vi "SP Handle Data Memory Enabling.vi"(7 "Memory Exists?":bool[](array[boolean]), 9 "CH Controls":T1[](array[typedef]) {"Reference" format="%#.2g"; "Display Data" items=["Data", "Memory", "Data/Memory"]; "Format" items=["Log Mag", "Phase", "Expanded Phase", "Delay", "Smith", "Polar", "Lin Mag", "SWR", "Loss", "Real", "Imaginary"]; "Scale" min=0.001 step=1.0 format="%#.2g"; "Position" min=0.0 max=10.0}, 10 "Parameters Measured":T4[](array[typedef]) {"Channel" min=1 max=99 step=1; "Parameter"."Stimulus Port" min=1 step=1; "Parameter"."Response Port" min=1 step=1}, 11 "Display Data Refs":refnum<vi>[](array[refnum])) -> ()   [LabVIEW 2011]
uses:
  TypeDefs/SP Parameter to Measure.ctl
  TypeDefs/SP Parameter.ctl
  TypeDefs/SP Calibration State.ctl
  TypeDefs/SP Measurement Format.ctl
  TypeDefs/SP Display Trace Controls.ctl
  TypeDefs/SP Display Format.ctl
  TypeDefs/SP Display Data.ctl
panel:
  # "Div"
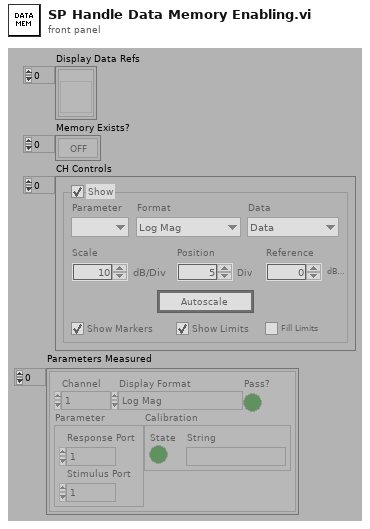
[diagram p1: front panel]
types:
  T1 = typedef "SP Display Trace Controls.ctl" = cluster{"Trace On":bool, "Measure":i32, "Format":T2, "Autoscale":bool, "Reference":dbl, "\nRefUnit":string, "Position":dbl, "Scale":dbl, "ScaleUnit":string, "LimitOn":bool, "LimitFill":bool, "Display Data":T3, "Show Markers":bool, "SXX":string}
  T2 = typedef "SP Display Format.ctl" = i32
  T3 = typedef "SP Display Data.ctl" = u16
  T4 = typedef "SP Parameter to Measure.ctl" = cluster{"Channel":i8, "Parameter":T5, "Calibration":T6, "Display Format":T7, "Pass?":bool}
  T5 = typedef "SP Parameter.ctl" = cluster{"Stimulus Port":i8, "Response Port":i8}
  T6 = typedef "SP Calibration State.ctl" = cluster{"State":bool, "String":string}
  T7 = typedef "SP Measurement Format.ctl" = enum32{"Log Mag", "Phase", "Delay", "Smith (R+jX)", "Polar (Re/Im)", "Linear Mag", "SWR", "Real", "Imaginary", "Smith (Lin/Phase)", "Smith (Log/Phase)", "Smith (Real/Imag)", "Smith (G+jB)", "Polar (Lin/Phase)", "Polar (Log/Phase)", "Expanded Phase", "Positive Phase", "Inverted Smith", "Unwrapped Phase", "Power Out", "Power In", "Linear Mag/Phase", "Log Mag/Phase", "Real/Imaginary"}
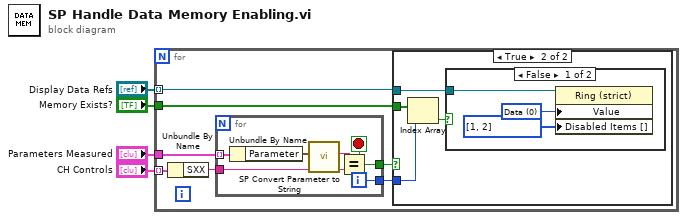
[diagram p0: block diagram]
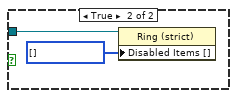
[diagram p3: hidden frame]
diagram:
  n1 = for {
    tunnel: "CH Controls" -> [w11] mode=indexing
    tunnel: "Memory Exists?" -> [w7]
    tunnel: "Display Data Refs" -> [w6] mode=indexing
    tunnel: "Parameters Measured" -> [w5]
    n2 = Unbundle By Name(w11) -> ("SXX"=w10:string)
    n3 = for {
      tunnel: w5 -> [w16] mode=indexing
      tunnel: w10 -> [w17]
      tunnel: [w14] -> w9
      tunnel: [w15] -> w8
      i -> [w15]
      stop <- w14 stop-if-true
      n4 = Unbundle By Name(w16) -> ("Parameter"=w13:T5)
      n5 = call "SP Convert Parameter to String.vi"("Parameter"=w13) -> ("Parameter String"=w12:string)  [unwired: 10 out]
      n6 = Equal?(x=w12, y=w17) -> (x = y?=w14:bool)
    }
    n7 = case shown="True" w9 {
      tunnel: w8 -> [_ w20]
      tunnel: w7 -> [_ w21]
      tunnel: w6 -> [_ w18]
      frame False {
      }
      frame True {
        n8 = Index Array(array=w21, index=w20) -> (element=w19:bool)
        n9 = case shown="False" w19 {
          tunnel: w18 -> [w24 w26]
          frame False {
            w22 = T3[] [1, 2] items=["Data", "Memory", "Data/Memory"]
            w23 = T3 0 items=["Data", "Memory", "Data/Memory"] ("Display Data")
            n10 = property class="Ring (strict)"(reference=w24, "Value"=w23, "Disabled Items []"=w22) -> ()  [unwired: 1 in, 2 out]
          }
          frame True {
            w25 = T3[] [] items=["Data", "Memory", "Data/Memory"]
            n11 = property class="Ring (strict)"(reference=w26, "Disabled Items []"=w25) -> ()  [unwired: 1 in, 2 out]
          }
        }
      }
    }
  }
